vi "IndexArray.vi"(9 "y":dbl, 10 "x":dbl, 11 "Array":dbl[](array[numeric])) -> (2 "?":dbl)   [LabVIEW 2017]
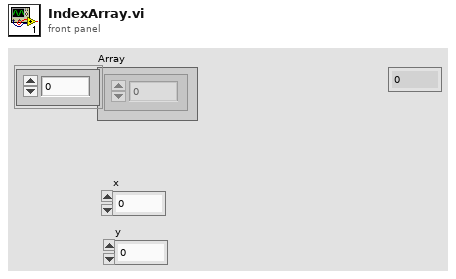
[diagram p1: front panel]
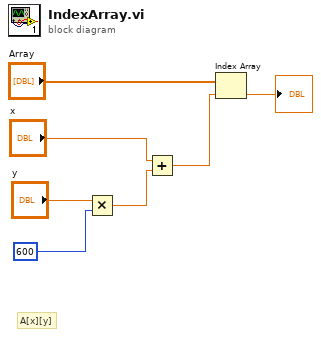
[diagram p0: block diagram]
diagram:
  # "A[x][y]"
  n1 = Multiply(x="y", y=600) -> (x*y=w5:dbl)
  n2 = Add(x="x", y=w5) -> (x+y=w2:dbl)
  n3 = Index Array(array="Array", index=w2) -> (element=→"?":dbl)
